vi "run.vi"(8 "error in (no error)":errorcluster, 11 "DL090216Display in":refnum<class "DisplayDL090216.lvclass">) -> (0 "error out":errorcluster, 3 "DL090216Display out":refnum<class "DisplayDL090216.lvclass">)   [LabVIEW 2010, in "DisplayDL090216.lvclass"]
uses:
  DisplayDL090216.lvclass
  common/clusters/range_offset_cluster.ctl
  common/enumerations/channel_display_colour_enum.ctl
  individual_channel_cluster.ctl
  main/labview_source/controls/undock_button.ctl
  action_enum.ctl
  <vilib>/vision/Image Controls.llb/IMAQ Image.ctl
  DisplayDL090216.lvclass/DisplayDL090216.ctl
  ImageProcessor/ImageProcessorDL090216RangeOffset/ImageProcessorDL090216RangeOffset/ImageProcessorDL090216RangeOffset.lvclass
  GenericDisplay/GenericDisplay/GenericDisplay.lvclass
  ImageProcessor/GenericImageProcessor/GenericImageProcessor/GenericImageProcessor.lvclass
  common/classes/Image/Image/colour_enum.ctl
  common/classes/ErrorController/ErrorController/class_data.vi
  common/classes/Image/Image/Image.lvclass
  common/classes/GenericComponent/GenericComponent/GenericComponent.lvclass
  common/classes/ErrorController/ErrorController/ErrorController.lvclass
panel:
  in  "button:undock_main_window":T1
  in  "button:undock":T1
  in  "button_configure":bool
  in  "channel tab":enum32{"Individual channels", "Debug"}(tab)
  in  "channel 3":T2
  in  "channel 2":T2
  in  "channel 1":T2
  out "statechart error":errorcluster
  out "event handling loop error":errorcluster
  out "first image received?":bool
  out "event handling loop counter":i32
  out "statemachine loop counter":i32
  out "current action":T4
  out "last trigger":T4
  in  "Tab Control":enum32{"Image", "Performance", "Extra"}(tab)=enum."Performance"
  in  "master range and offset":T5={"range"=0.5, "offset"=0.5} {"offset" min=0.0 max=1.0 step=0.0010000000474974513 scale=0.0..1.0; "range" min=0.0 max=1.0 step=0.0010000000474974513 scale=0.0..1.0}
  in  "optimise":bool
  in  "adjust range/offset button":bool
  in  "channel colours":T6[](array[typedef])=[enum."red", enum."green", enum."blue", enum."red"]
  in  "elements in queue":i32
  in  "maximum resolution":i32=256 min=0 max=512
  in  "maximum update rate":dbl[unit]=10.0 min=0.0
  in  "button:show_histogram?":bool caption="show histogram"
  in  "x scaling":dbl(slide)=1.0 min=0.05 max=20.0 step=0.01 scale=0.05..20.0
  in  "rotated by":dbl[unit]
  in  "enable x middle line?":bool
  in  "enable y middle line?":bool
  in  "enable scale bar?":bool
  in  "flipped?":bool
  in  "zero rotation button":bool
  in  "averaging":i32=1 min=1 max=100 step=1
  in  "stop":bool
  out "main display":T3(plugin-control)
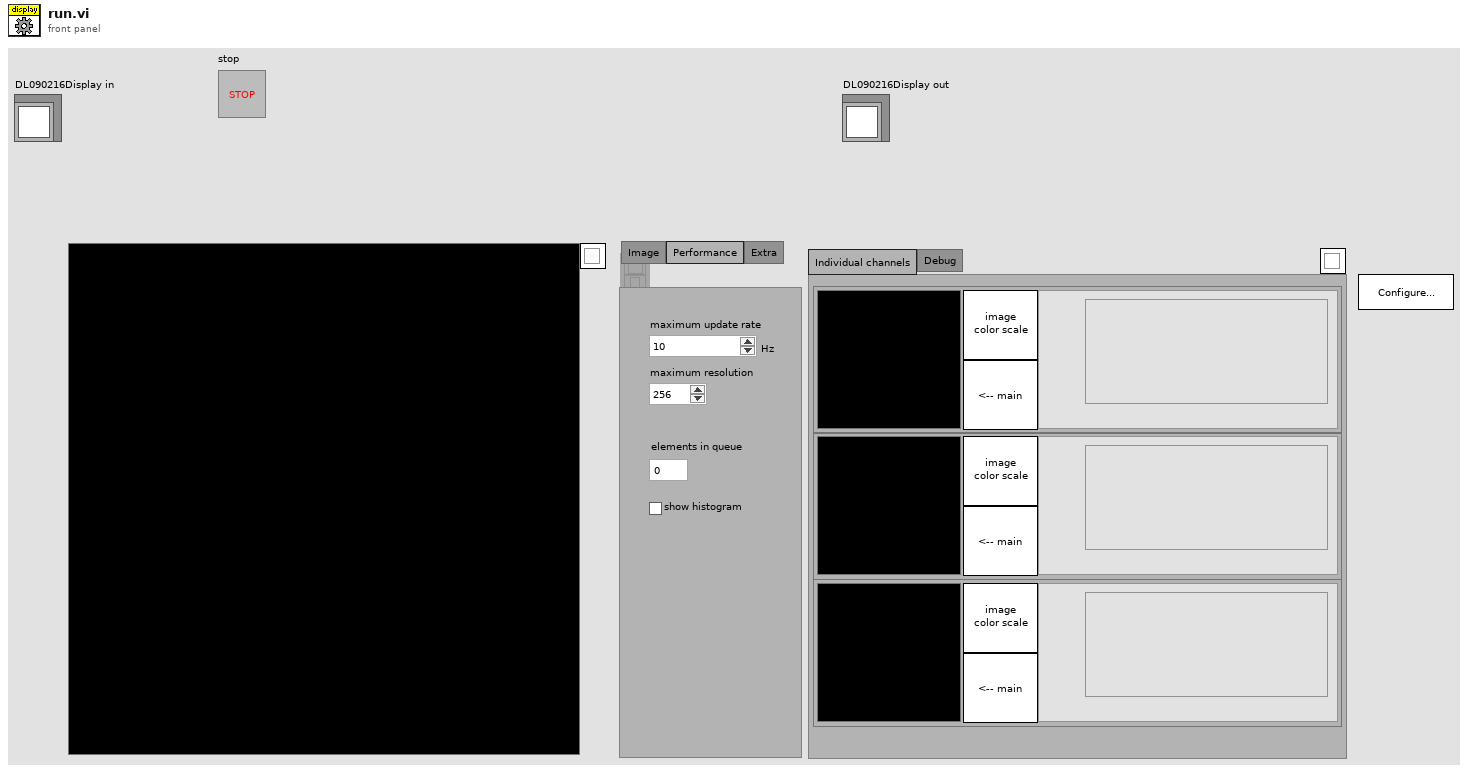
[diagram p1: front panel]
types:
  T1 = typedef "undock_button.ctl" = bool
  T2 = typedef "DisplayDL090216.lvclass/individual_channel_cluster.ctl" = cluster{"Image":T3, "histogram out":cluster{i32, u32}[], "button:color scale":bool, "button:set as main image":bool}
  T3 = typedef "IMAQ Image.ctl" = refnum<image>
  T4 = typedef "DisplayDL090216.lvclass/action_enum.ctl" = enum16{"NULL", "initialise", "experiment started", "experiment stopped", "terminate", "fetch", "process", "display", "register as observer"}
  T5 = typedef "range_offset_cluster.ctl" = cluster{"range":dbl, "offset":dbl}
  T6 = typedef "channel_display_colour_enum.ctl" = enum16{"none", "red", "green", "blue", "grey scale", "custom"}
  T7 = typedef "main_trigger_enum.ctl" = enum16{"NULL", "initialise", "terminate", "start", "stop", "change objective", "change experimentController", "change imagingMode", "save notebook", "started saving", "finished saving", "expCtr ready", "expCtr missing", "imgMd ready", "imgMd missing", "scanHd ready", "scanHd missing", "DAQ ready", "DAQ missing", "imgAsm ready", "imgAsm missing", "dataColl ready", "dataColl missing", "display ready", "display missing", "analysr ready", "analysr missing", "instrmnt ready", "instrmnt missing", "stimltr ready", "stimltr missing", "stage ready", "stage missing"}
  T8 = enum8{"Enabled", "Disabled", "Disabled and Grayed Out"}
  T9 = typedef "Image.lvclass/colour_enum.ctl" = enum16{"none", "red", "green", "blue", "grey scale", "custom"}
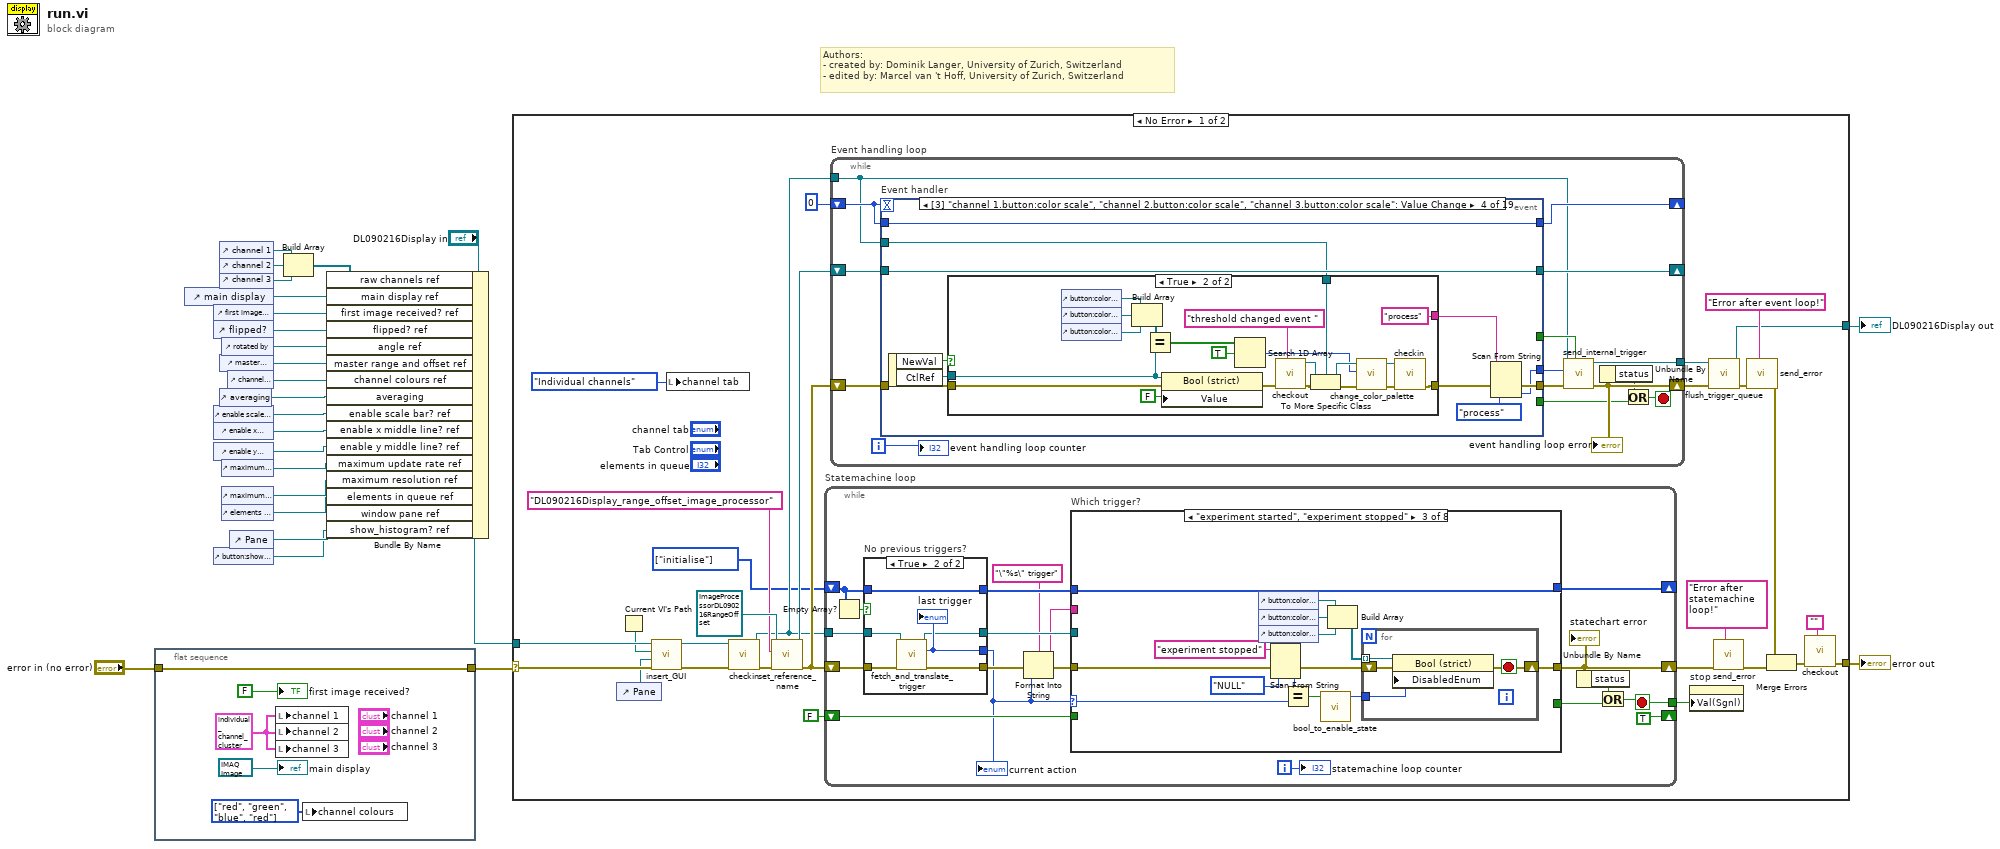
[diagram p0: block diagram]
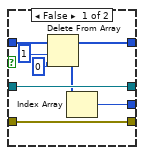
[diagram p2: hidden frame]
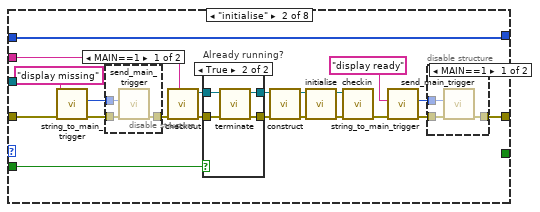
[diagram p4: hidden frame]
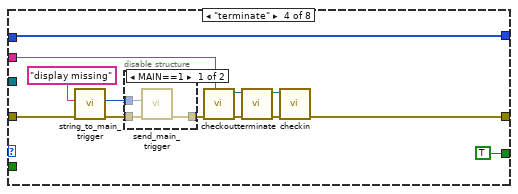
[diagram p8: hidden frame]
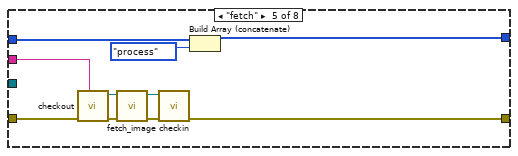
[diagram p10: hidden frame]
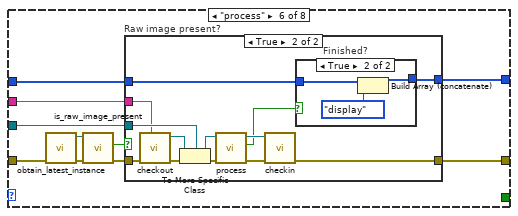
[diagram p11: hidden frame]
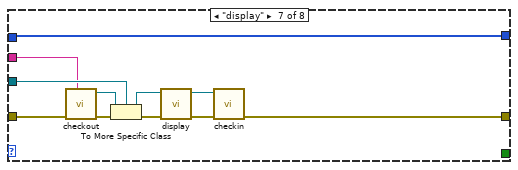
[diagram p14: hidden frame]
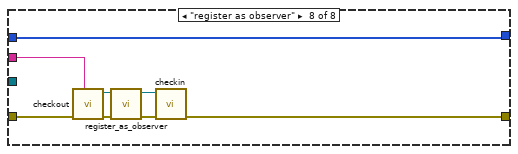
[diagram p15: hidden frame]
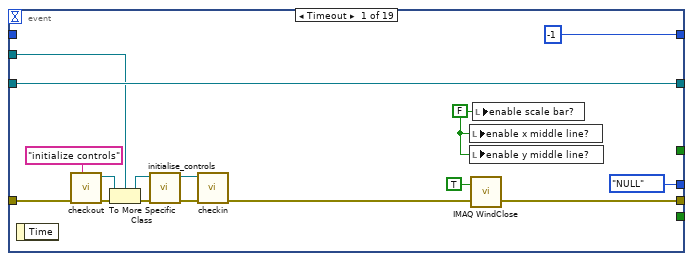
[diagram p16: hidden frame]
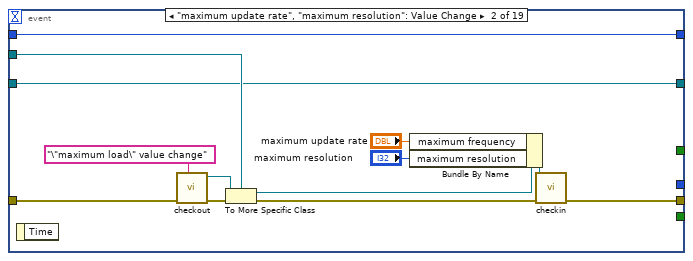
[diagram p17: hidden frame]
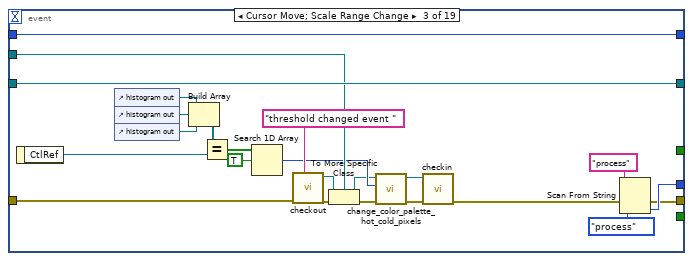
[diagram p18: hidden frame]
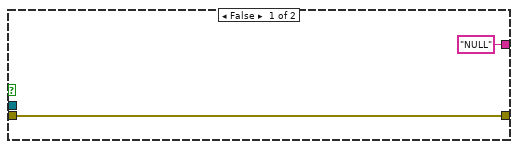
[diagram p19: hidden frame]
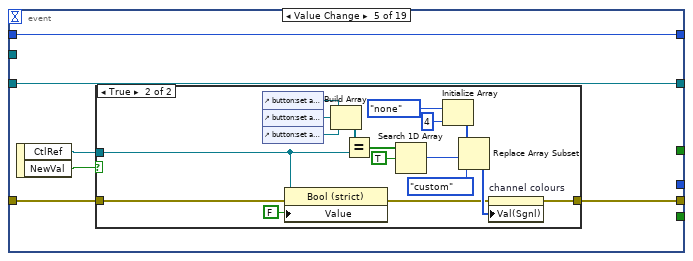
[diagram p20: hidden frame]
diagram:
  # "Authors: \n- created by: Dominik Langer, University of Zurich, Switzerland\n- edited by: Marcel van 't Hoff, University of Zurich, Switzerland"
  n1 = flat-sequence {
    tunnel: "error in (no error)" -> [w30]
    tunnel: [w30] -> w6
    frame #0 {
      w26 = T6[] [enum."red", enum."green", enum."blue", enum."red"] items=["none", "red", "green", "blue", "grey scale", "custom"] ("channel colours")
      w27 = T2 {"Image"=refnum, "histogram out"=[], "button:color scale"=FALSE, "button:set as main image"=FALSE} ("channel 1")
      n2 = local write "channel 1"(w27) -> ()
      n3 = local write "channel 2"(w27) -> ()
      n4 = local write "channel 3"(w27) -> ()
      n5 = local write "channel colours"(w26) -> ()
      "first image received?" <- FALSE
      "main display" <- T3 refnum ("main display")
    }
  }
  n6 = control-ref of="main display"() -> (w21:refnum<vi>)
  n7 = control-ref of="first image received?"() -> (w3:refnum<vi>)
  n8 = control-ref of="flipped?"() -> (w20:refnum<vi>)
  n9 = control-ref of="enable scale bar?"() -> (w16:refnum<vi>)
  n10 = control-ref of="enable x middle line?"() -> (w15:refnum<vi>)
  n11 = control-ref of="enable y middle line?"() -> (w14:refnum<vi>)
  n12 = control-ref of="button:show_histogram?"() -> (w2:refnum<vi>)
  n13 = control-ref of="channel 1"() -> (w8:refnum<vi>)
  n14 = control-ref of="channel 2"() -> (w9:refnum<vi>)
  n15 = control-ref of="channel 3"() -> (w10:refnum<vi>)
  n16 = control-ref of="master range and offset"() -> (w17:refnum<vi>)
  n17 = control-ref of="averaging"() -> (w1:refnum<vi>)
  n18 = control-ref of="rotated by"() -> (w19:refnum<vi>)
  n19 = control-ref of="maximum update rate"() -> (w5:refnum<vi>)
  n20 = control-ref of="maximum resolution"() -> (w13:refnum<vi>)
  n21 = control-ref of="elements in queue"() -> (w12:refnum<vi>)
  n22 = control-ref of="channel colours"() -> (w18:refnum<vi>)
  n23 = control-ref of="Pane"() -> (w11:refnum<vi>)
  n24 = Build Array(w8, w9, w10) -> (w4:refnum<vi>[])
  n25 = Bundle By Name(cluster="DL090216Display in", "raw channels ref"=w4, "main display ref"=w21, "first image received? ref"=w3, "flipped? ref"=w20, "angle ref"=w19, "master range and offset ref"=w17, "channel colours ref"=w18, "averaging"=w1, "enable scale bar? ref"=w16, "enable x middle line? ref"=w15, "enable y middle line? ref"=w14, "maximum update rate ref"=w5, "maximum resolution ref"=w13, "elements in queue ref"=w12, "window pane ref"=w11, "show_histogram? ref"=w2) -> (w22:refnum<class "DisplayDL090216.lvclass">)
  n26 = case shown="No Error" w6 {
    selector: w6 -> [w51 w575]
    tunnel: [w43 w575] -> w25
    tunnel: [w41 w574] -> w24
    tunnel: w22 -> [w50 w574]
    frame No Error {
      w34 = T4[] [enum."initialise"] items=["NULL", "initialise", "experiment started", "experiment stopped", "terminate", "fetch", "process", "display", "register as observer"]
      n27 = control-ref of="Pane"() -> (w48:refnum<vi>)
      n28 = Current VI's Path() -> (path=w49:path)
      n29 = call-dynamic "insert_GUI.vi"("error in (no error)"=w51, "Pane"=w48, "VI path"=w49, "GenericComponent in"=w50) -> ("error out"=w33:errorcluster, "GenericComponent out"=w36:refnum<class "DisplayDL090216.lvclass">)  [unwired: 6 in]
      n30 = local write "channel tab"(enum32{"Individual channels", "Debug"}."Individual channels" ("channel tab")) -> ()
      n31 = call-dynamic "checkin.vi"("error in (no error)"=w33, "GenericDisplay in"=w36) -> ("error out"=w53:errorcluster, "GenericDisplay out"=w37:refnum<class "DisplayDL090216.lvclass">)  [unwired: 8 in]
      n32 = call "set_reference_name.vi"("error in (no error)"=w53, "reference name"="DL090216Display_range_offset_image_processor", "GenericPlugin.lvclass in"=refnum<class "ImageProcessorDL090216RangeOffset.lvclass"> refnum ("ImageProcessorDL090216RangeOffset.lvclass")) -> ("error out"=w38:errorcluster, "GenericPlugin.lvclass out"=w52:refnum<class "ImageProcessorDL090216RangeOffset.lvclass">)  [unwired: 7 in]
      n33 = while "Statemachine loop" {
        shift-right: [w75] -> w32
        shift-left: w38 -> [w76]
        tunnel: [w72] -> w57
        tunnel: w37 -> [w77]
        shift-right: [w71] -> _
        shift-left: w34 -> [w68]
        shift-right: [TRUE] -> _
        shift-left: FALSE -> [w66]
        i -> [w78]
        stop <- w72 stop-if-true
        n34 = Empty Array?(array=w68) -> (empty?=w67:bool)
        n35 = case "No previous triggers?" shown="True" w67 {
          tunnel: w77 -> [w85 w92]
          tunnel: w76 -> [w86 w91]
          tunnel: [w86 w90] -> w64
          tunnel: [w79 w89] -> w63
          tunnel: w68 -> [w84 w88]
          tunnel: [w81 w88] -> w70
          tunnel: [w85 w87] -> w69
          frame False {
            n36 = Delete From Array(array=w84, length=1, index=0) -> (deleted portion=w80:T4[], array with subset deleted=w81:T4[])
            n37 = Index Array(array=w80) -> (element=w79:T4)  [unwired: 1 in]
          }
          frame True {
            n38 = call-dynamic "fetch_and_translate_trigger.vi"("error in (no error)"=w91, "DisplayDL090216 in"=w92) -> ("error out"=w90:errorcluster, "internal trigger"=w89:T4, "DisplayDL090216 out"=w87:refnum<class "DisplayDL090216.lvclass">)  [unwired: 6 in, 1 out]
            "last trigger" <- w89
          }
        }
        "current action" <- w63
        n39 = Format Into String(format string="\"%s\" trigger", error in=w64, w63) -> (resulting string=w61:string, error out=w62:errorcluster)  [unwired: 1 in]
        n40 = case "Which trigger?" shown="\"experiment started\", \"experiment stopped\"" w63 {
          selector: w63 -> [_ _ w137 _ _ _ _ _]
          tunnel: w62 -> [w94 w97 w131 w151 w170 w180 w208 w218]
          tunnel: [w94 w111 w138 w157 w169 w177 w207 w217] -> w75
          tunnel: [_ _ _ TRUE _ _ _ _] -> w74
          tunnel: [w93 w110 w143 w153 w167 w183 w206 w216] -> w71
          tunnel: w70 -> [w93 w110 w143 w153 w166 w184 w206 w216]
          tunnel: w69 -> [_ _ _ _ _ w178 w205 _]
          tunnel: w66 -> [_ w105 _ _ _ _ _ _]
          tunnel: w61 -> [_ w104 _ w152 w165 w175 w204 w215]
          frame "NULL", Default {
          }
          frame "initialise" {
            n41 = call "string_to_main_trigger.vi"("error in (no error)"=w97, "trigger string"="display missing") -> ("error out"=w99:errorcluster, "main trigger"=w98:T7)  [unwired: 8 in]
            n42 = disable-structure shown="MAIN==1" {
              disable-tunnel: w99 -> [w118 w119]
              disable-tunnel: [w117 w119] -> w96
              disable-tunnel: w98 -> [w116 _]
              frame condition #0 {
                n43 = call "send_main_trigger.vi"("error in (no error)"=w118, "trigger"=w116) -> ("error out"=w117:errorcluster)  [unwired: 9 in]
              }
              frame condition #1 (active) {
              }
            }
            n44 = call "checkout.vi"("locked by?"=w104, "error in (no error)"=w96) -> ("error out"=w109:errorcluster, "GenericDisplay out"=w108:refnum<class "GenericDisplay.lvclass">)  [unwired: 8 out]
            n45 = case "Already running?" shown="True" w105 {
              tunnel: w109 -> [w124 w129]
              tunnel: w108 -> [w125 w128]
              tunnel: [w125 w127] -> w107
              tunnel: [w124 w126] -> w106
              frame False {
              }
              frame True {
                n46 = call-dynamic "terminate.vi"("error in (no error)"=w129, "GenericPlugin in"=w128) -> ("error out"=w126:errorcluster, "GenericPlugin out"=w127:refnum<class "GenericDisplay.lvclass">)  [unwired: 8 in]
              }
            }
            n47 = call-dynamic "construct.vi"("error in (no error)"=w106, "GenericPlugin in"=w107) -> ("error out"=w115:errorcluster, "GenericPlugin out"=w114:refnum<class "GenericDisplay.lvclass">)  [unwired: 2 in, 6 out]
            n48 = call-dynamic "initialise.vi"("error in (no error)"=w115, "GenericPlugin in"=w114) -> ("error out"=w113:errorcluster, "GenericPlugin out"=w112:refnum<class "GenericDisplay.lvclass">)  [unwired: 8 out]
            n49 = call-dynamic "checkin.vi"("error in (no error)"=w113, "GenericDisplay in"=w112) -> ("error out"=w101:errorcluster)  [unwired: 8 in, 1 out]
            n50 = call "string_to_main_trigger.vi"("error in (no error)"=w101, "trigger string"="display ready") -> ("error out"=w100:errorcluster, "main trigger"=w102:T7)  [unwired: 8 in]
            n51 = disable-structure shown="MAIN==1" {
              disable-tunnel: w100 -> [w122 w123]
              disable-tunnel: [w121 w123] -> w111
              disable-tunnel: w102 -> [w120 _]
              frame condition #0 {
                n52 = call "send_main_trigger.vi"("error in (no error)"=w122, "trigger"=w120) -> ("error out"=w121:errorcluster)  [unwired: 9 in]
              }
              frame condition #1 (active) {
              }
            }
          }
          frame "experiment started", "experiment stopped" {
            n53 = control-ref of="button:color scale"() -> (w140:refnum<vi>)
            n54 = control-ref of="button:color scale"() -> (w141:refnum<vi>)
            n55 = control-ref of="button:color scale"() -> (w142:refnum<vi>)
            n56 = Scan From String(input string="experiment stopped", error in=w131, default 1=action_enum."NULL" ("y")) -> (error out=w135:errorcluster, output 1=w133:T4)  [unwired: 2 in, 2 out]
            n57 = Equal?(x=w133, y=w137) -> (x = y?=w130:bool)
            n58 = call "bool_to_enable_state.vi"("boolean in"=w130) -> ("enabled status out"=w132:T8)  [unwired: 4 in]
            n59 = Build Array(w140, w141, w142) -> (w139:refnum<vi>[])
            n60 = for {
              tunnel: w139 -> [w147] mode=indexing
              shift-right: [w145] -> w138
              shift-left: w135 -> [w146]
              tunnel: w132 -> [w144]
              stop <- w145 stop-if-true
              n61 = property class="Bool (strict)"(reference=w147, error in=w146, "DisabledEnum"=w144) -> (error out=w145:errorcluster)  [unwired: 1 out]
            }
          }
          frame "terminate" {
            n62 = call "string_to_main_trigger.vi"("error in (no error)"=w151, "trigger string"="display missing") -> ("error out"=w150:errorcluster, "main trigger"=w148:T7)  [unwired: 8 in]
            n63 = disable-structure shown="MAIN==1" {
              disable-tunnel: w150 -> [w163 w164]
              disable-tunnel: [w162 w164] -> w154
              disable-tunnel: w148 -> [w161 _]
              frame condition #0 {
                n64 = call "send_main_trigger.vi"("error in (no error)"=w163, "trigger"=w161) -> ("error out"=w162:errorcluster)  [unwired: 9 in]
              }
              frame condition #1 (active) {
              }
            }
            n65 = call "checkout.vi"("locked by?"=w152, "error in (no error)"=w154) -> ("error out"=w156:errorcluster, "GenericDisplay out"=w158:refnum<class "GenericDisplay.lvclass">)  [unwired: 8 out]
            n66 = call-dynamic "terminate.vi"("error in (no error)"=w156, "GenericPlugin in"=w158) -> ("error out"=w155:errorcluster, "GenericPlugin out"=w159:refnum<class "GenericDisplay.lvclass">)  [unwired: 8 out]
            n67 = call-dynamic "checkin.vi"("error in (no error)"=w155, "GenericDisplay in"=w159) -> ("error out"=w157:errorcluster)  [unwired: 8 in, 1 out]
          }
          frame "fetch" {
            n68 = call "checkout.vi"("locked by?"=w165, "error in (no error)"=w170) -> ("error out"=w173:errorcluster, "GenericDisplay out"=w172:refnum<class "GenericDisplay.lvclass">)  [unwired: 8 out]
            n69 = call-dynamic "fetch_image.vi"("error in (no error)"=w173, "GenericToplevelComponent in"=w172) -> ("error out"=w174:errorcluster, "GenericToplevelComponent out"=w171:refnum<class "GenericDisplay.lvclass">)  [unwired: 4 in, 4 out]
            n70 = call-dynamic "checkin.vi"("error in (no error)"=w174, "GenericDisplay in"=w171) -> ("error out"=w169:errorcluster)  [unwired: 8 in, 1 out]
            n71 = Build Array (concatenate)(w166, action_enum."process" ("last trigger")) -> (w167:T4[])
          }
          frame "process" {
            n72 = call "obtain_latest_instance.vi"("error in (no error)"=w180) -> ("error out"=w182:errorcluster, "GenericDisplay out"=w181:refnum<class "GenericDisplay.lvclass">)  [unwired: 1 in, 8 out]
            n73 = call-dynamic "is_raw_image_present.vi"("error in (no error)"=w182, "GenericDisplay in"=w181) -> ("error out"=w179:errorcluster, "raw image present?"=w176:bool)  [unwired: 8 out]
            n74 = case "Raw image present?" shown="True" w176 {
              tunnel: w184 -> [w186 w199]
              tunnel: [w186 w198] -> w183
              tunnel: w179 -> [w185 w192]
              tunnel: w178 -> [_ w191]
              tunnel: [w185 w189] -> w177
              tunnel: w175 -> [_ w188]
              frame False {
              }
              frame True {
                n75 = call "checkout.vi"("locked by?"=w188, "error in (no error)"=w192) -> ("error out"=w197:errorcluster, "GenericDisplay out"=w196:refnum<class "GenericDisplay.lvclass">)  [unwired: 8 out]
                n76 = To More Specific Class(target class=w191, reference=w196, error in=w197) -> (specific class reference=w190:refnum<class "DisplayDL090216.lvclass">, error out=w195:errorcluster)
                n77 = call-dynamic "process.vi"("error in (no error)"=w195, "DL090216Display in"=w190) -> ("error out"=w194:errorcluster, "finished?"=w187:bool, "DL090216Display out"=w193:refnum<class "DisplayDL090216.lvclass">)  [unwired: 7 out]
                n78 = call-dynamic "checkin.vi"("error in (no error)"=w194, "GenericDisplay in"=w193) -> ("error out"=w189:errorcluster)  [unwired: 8 in, 1 out]
                n79 = case "Finished?" shown="True" w187 {
                  tunnel: w199 -> [w200 w203]
                  tunnel: [w200 w201] -> w198
                  frame False {
                  }
                  frame True {
                    n80 = Build Array (concatenate)(w203, action_enum."display" ("last trigger")) -> (w201:T4[])
                  }
                }
              }
            }
          }
          frame "display" {
            n81 = call "checkout.vi"("locked by?"=w204, "error in (no error)"=w208) -> ("error out"=w214:errorcluster, "GenericDisplay out"=w213:refnum<class "GenericDisplay.lvclass">)  [unwired: 8 out]
            n82 = To More Specific Class(target class=w205, reference=w213, error in=w214) -> (specific class reference=w209:refnum<class "DisplayDL090216.lvclass">, error out=w210:errorcluster)
            n83 = call-dynamic "display.vi"("error in (no error)"=w210, "DL090216Display in"=w209) -> ("error out"=w212:errorcluster, "DL090216Display out"=w211:refnum<class "DisplayDL090216.lvclass">)  [unwired: 8 out]
            n84 = call-dynamic "checkin.vi"("error in (no error)"=w212, "GenericDisplay in"=w211) -> ("error out"=w207:errorcluster)  [unwired: 8 in, 1 out]
          }
          frame "register as observer" {
            n85 = call "checkout.vi"("locked by?"=w215, "error in (no error)"=w218) -> ("error out"=w220:errorcluster, "GenericDisplay out"=w222:refnum<class "GenericDisplay.lvclass">)  [unwired: 8 in]
            n86 = call-dynamic "register_as_observer.vi"("error in (no error)"=w220, "GenericToplevelComponent in"=w222) -> ("error out"=w219:errorcluster, "GenericToplevelComponent out"=w221:refnum<class "GenericDisplay.lvclass">)  [unwired: 8 in]
            n87 = call-dynamic "checkin.vi"("error in (no error)"=w219, "GenericDisplay in"=w221) -> ("error out"=w217:errorcluster)  [unwired: 8 in, 1 out]
          }
        }
        "statechart error" <- w75
        n88 = Unbundle By Name(w75) -> ("status"=w73:bool)
        n89 = Or(x=w73, y=w74) -> (x .or. y?=w72:bool)
        "statemachine loop counter" <- w78
      }
      n90 = while "Event handling loop" {
        shift-right: [w227] -> w42
        shift-left: w38 -> [w237]
        shift-right: [w235] -> _
        shift-left: 0 -> [w236]
        shift-right: [w233] -> _
        shift-left: w52 -> [w232]
        tunnel: w37 -> [w228]
        tunnel: [w230] -> w40
        i -> [w234]
        stop <- w224 stop-if-true
        n91 = event "Event handler" shown="[3] \"channel 1.button:color scale\", \"channel 2.button:color scale\", \"channel 3.button:color scale\": Value Change" {
          selector: _ -> [_ _ _ _ _ _ _ _ _ _ _ _ _ _ _ _ _ _ _]
          dyn-events: _ -> [_ _ _ _ _ _ _ _ _ _ _ _ _ _ _ _ _ _ _]
          timeout: w236 -> [_ _ _ _ _ _ _ _ _ _ _ _ _ _ _ _ _ _ _]
          tunnel: w237 -> [w249 w264 w288 w297 w328 w364 w378 w384 w401 w420 w426 w446 w453 w474 w500 w516 w521 w555 w568]
          tunnel: [w240 w263 w267 w293 w327 w349 w374 w383 w392 w419 w425 w431 w452 w465 w488 w510 w524 w541 w561] -> w231
          tunnel: [-1 w266 w290 w301 w330 w361 w380 w387 w403 w423 w429 w450 w463 w486 w504 w518 w539 w559 w573] -> w235
          tunnel: w236 -> [_ w266 w290 w301 w330 w361 w380 w387 w403 w423 w429 w450 w463 w486 w504 w518 w539 w559 w573]
          tunnel: [_ _ _ _ _ _ _ _ _ _ TRUE _ _ _ _ _ _ _ _] -> w225
          tunnel: w228 -> [w245 w259 w287 w299 _ w359 w371 w385 w398 _ _ w445 w458 w475 _ w508 w538 w554 w571]
          tunnel: [w251 w255 w289 w300 w329 w366 w379 w386 w402 w422 w427 w435 w455 w476 w493 w509 w528 w545 w565] -> w233
          tunnel: w232 -> [w251 w255 w289 w300 w329 w366 w379 w386 w402 w422 w427 w435 w454 w476 w493 w509 w528 w545 w565]
          tunnel: [_ _ _ _ _ _ _ _ _ _ _ _ TRUE _ _ _ _ _ _] -> w229
          tunnel: [action_enum."NULL" ("trigger") _ w269 w292 _ w351 _ _ _ _ _ w430 _ w464 w487 _ w523 w540 w560] -> w223
          event Timeout {
            w252 = FALSE
            n92 = event-data() -> ()  [unwired: 2 out]
            n93 = call "checkout.vi"("locked by?"="initialize controls", "error in (no error)"=w249) -> ("error out"=w250:errorcluster, "GenericDisplay out"=w246:refnum<class "GenericDisplay.lvclass">)  [unwired: 8 out]
            n94 = To More Specific Class(target class=w245, reference=w246, error in=w250) -> (specific class reference=w244:refnum<class "DisplayDL090216.lvclass">, error out=w248:errorcluster)
            n95 = call-dynamic "initialise_controls.vi"("error in (no error)"=w248, "DL090216Display in"=w244) -> ("error out"=w247:errorcluster, "DL090216Display out"=w243:refnum<class "DisplayDL090216.lvclass">)  [unwired: 8 out]
            n96 = call-dynamic "checkin.vi"("error in (no error)"=w247, "GenericDisplay in"=w243) -> ("error out"=w241:errorcluster)  [unwired: 8 in, 1 out]
            n97 = local write "enable x middle line?"(w252) -> ()
            n98 = local write "enable y middle line?"(w252) -> ()
            n99 = call "IMAQ WindClose"("Close All Windows (False)"=TRUE, "error in (no error)"=w241) -> ("error out"=w240:errorcluster)  [unwired: 4 in]
            n100 = local write "enable scale bar?"(w252) -> ()
          }
          event "maximum update rate", "maximum resolution": Value Change {
            n101 = event-data() -> ()  [unwired: 2 out]
            n102 = call "checkout.vi"("locked by?"="\"maximum load\" value change", "error in (no error)"=w264) -> ("error out"=w262:errorcluster, "GenericDisplay out"=w260:refnum<class "GenericDisplay.lvclass">)  [unwired: 8 in]
            n103 = To More Specific Class(target class=w259, reference=w260, error in=w262) -> (specific class reference=w258:refnum<class "DisplayDL090216.lvclass">, error out=w261:errorcluster)
            n104 = Bundle By Name(cluster=w258, "maximum frequency"="maximum update rate", "maximum resolution"="maximum resolution") -> (w257:refnum<class "DisplayDL090216.lvclass">)
            n105 = call-dynamic "checkin.vi"("error in (no error)"=w261, "GenericDisplay in"=w257) -> ("error out"=w263:errorcluster)  [unwired: 8 in, 1 out]
          }
          event Cursor Move; Scale Range Change {
            n106 = event-data() -> ("CtlRef"=w286:refnum<vi>)  [unwired: 1 out]
            n107 = control-ref of="histogram out"() -> (w282:refnum<vi>)
            n108 = control-ref of="histogram out"() -> (w281:refnum<vi>)
            n109 = control-ref of="histogram out"() -> (w280:refnum<vi>)
            n110 = Build Array(w282, w281, w280) -> (w279:refnum<vi>[])
            n111 = Equal?(x=w279, y=w286) -> (x = y?=w278:bool[])
            n112 = Search 1D Array(1D array=w278, element=TRUE) -> (index of element=w276:i32)  [unwired: 1 in]
            n113 = call "checkout.vi"("locked by?"="threshold changed event ", "error in (no error)"=w288) -> ("error out"=w285:errorcluster, "GenericDisplay out"=w284:refnum<class "GenericDisplay.lvclass">)  [unwired: 8 out]
            n114 = To More Specific Class(target class=w287, reference=w284, error in=w285) -> (specific class reference=w275:refnum<class "DisplayDL090216.lvclass">, error out=w273:errorcluster)
            n115 = call-dynamic "change_color_palette_hot_cold_pixels.vi"("error in (no error)"=w273, "raw channel index"=w276, "DisplayDL090216 in"=w275) -> ("error out"=w272:errorcluster, "DisplayDL090216 out"=w274:refnum<class "DisplayDL090216.lvclass">)  [unwired: 7 in]
            n116 = call-dynamic "checkin.vi"("error in (no error)"=w272, "GenericDisplay in"=w274) -> ("error out"=w268:errorcluster)  [unwired: 8 in, 1 out]
            n117 = Scan From String(input string="process", error in=w268, default 1=action_enum."process" ("trigger")) -> (error out=w267:errorcluster, output 1=w269:T4)  [unwired: 2 in, 2 out]
          }
          event Value Change {
            n118 = event-data() -> ("NewVal"=w296:bool, "CtlRef"=w298:refnum<vi>)  [unwired: 1 out]
            n119 = case shown="True" w296 {
              tunnel: [w303 w324] -> w294
              tunnel: w299 -> [_ w323]
              tunnel: w298 -> [_ w308]
              tunnel: w297 -> [w303 w307]
              tunnel: ["NULL" "process"] -> w291
              frame False {
              }
              frame True {
                n120 = control-ref of="button:color scale"() -> (w319:refnum<vi>)
                n121 = control-ref of="button:color scale"() -> (w318:refnum<vi>)
                n122 = control-ref of="button:color scale"() -> (w317:refnum<vi>)
                n123 = Build Array(w319, w318, w317) -> (w316:refnum<vi>[])
                n124 = Equal?(x=w316, y=w308) -> (x = y?=w315:bool[])
                n125 = property class="Bool (strict)"(reference=w308, error in=w307, "Value"=FALSE) -> (error out=w306:errorcluster)  [unwired: 1 out]
                n126 = Search 1D Array(1D array=w315, element=TRUE) -> (index of element=w309:i32)  [unwired: 1 in]
                n127 = call "checkout.vi"("locked by?"="threshold changed event ", "error in (no error)"=w306) -> ("error out"=w322:errorcluster, "GenericDisplay out"=w321:refnum<class "GenericDisplay.lvclass">)  [unwired: 8 out]
                n128 = To More Specific Class(target class=w323, reference=w321, error in=w322) -> (specific class reference=w313:refnum<class "DisplayDL090216.lvclass">, error out=w311:errorcluster)
                n129 = call-dynamic "change_color_palette.vi"("error in (no error)"=w311, "raw channel index"=w309, "DisplayDL090216 in"=w313) -> ("error out"=w310:errorcluster, "DisplayDL090216 out"=w312:refnum<class "DisplayDL090216.lvclass">)  [unwired: 7 in]
                n130 = call-dynamic "checkin.vi"("error in (no error)"=w310, "GenericDisplay in"=w312) -> ("error out"=w324:errorcluster)  [unwired: 8 in, 1 out]
              }
            }
            n131 = Scan From String(input string=w291, error in=w294, default 1=action_enum."process" ("trigger")) -> (error out=w293:errorcluster, output 1=w292:T4)  [unwired: 2 in, 2 out]
          }
          event Value Change {
            n132 = event-data() -> ("CtlRef"=w326:refnum<vi>, "NewVal"=w325:bool)  [unwired: 1 out]
            n133 = case shown="True" w325 {
              tunnel: w328 -> [w331 w334]
              tunnel: [w331 w348] -> w327
              tunnel: w326 -> [_ w335]
              frame False {
              }
              frame True {
                n134 = control-ref of="button:set as main image"() -> (w346:refnum<vi>)
                n135 = control-ref of="button:set as main image"() -> (w347:refnum<vi>)
                n136 = control-ref of="button:set as main image"() -> (w345:refnum<vi>)
                n137 = property class="Bool (strict)"(reference=w335, error in=w334, "Value"=FALSE) -> (error out=w333:errorcluster)  [unwired: 1 out]
                n138 = Build Array(w346, w347, w345) -> (w344:refnum<vi>[])
                n139 = Equal?(x=w344, y=w335) -> (x = y?=w343:bool[])
                n140 = Search 1D Array(1D array=w343, element=TRUE) -> (index of element=w338:i32)  [unwired: 1 in]
                n141 = Initialize Array(channel_display_colour_enum."none" ("channel x"), 4 ("element")) -> (w339:T6[])
                n142 = Replace Array Subset(array=w339, new element=channel_display_colour_enum."custom" ("new element/subarray"), index=w338) -> (w336:T6[])
                n143 = property on="channel colours" class="Arr (strict)"(error in=w333, "Val(Sgnl)"=w336) -> (error out=w348:errorcluster)  [unwired: 1 in, 1 out]
              }
            }
          }
          event "button_configure": Value Change {
            n144 = event-data() -> ()  [unwired: 4 out]
            n145 = call "checkout.vi"("locked by?"=" \"button_configure\" value change" ("string"), "error in (no error)"=w364) -> ("error out"=w365:errorcluster, "GenericDisplay out"=w363:refnum<class "GenericDisplay.lvclass">)  [unwired: 8 out]
            n146 = call-dynamic "configure.vi"("error in (no error)"=w365, "GenericPlugin in"=w363) -> ("error out"=w355:errorcluster, "GenericPlugin out"=w360:refnum<class "GenericDisplay.lvclass">)  [unwired: 8 in]
            n147 = To More Specific Class(target class=w359, reference=w360, error in=w355) -> (specific class reference=w358:refnum<class "DisplayDL090216.lvclass">, error out=w357:errorcluster)
            n148 = call-dynamic "set_histogram_enabled.vi"("error in (no error)"=w357, "DisplayDL090216 in"=w358) -> ("error out"=w354:errorcluster, "DisplayDL090216 out"=w356:refnum<class "DisplayDL090216.lvclass">)  [unwired: 8 in]
            n149 = call-dynamic "checkin.vi"("error in (no error)"=w354, "GenericDisplay in"=w356) -> ("error out"=w350:errorcluster)  [unwired: 8 in, 1 out]
            n150 = Scan From String(input string="initialise", error in=w350, default 1=action_enum."process" ("trigger")) -> (error out=w349:errorcluster, output 1=w351:T4)  [unwired: 2 in, 2 out]
          }
          event "button:show_histogram?": Value Change {
            n151 = event-data() -> ()  [unwired: 4 out]
            n152 = call "checkout.vi"("locked by?"=" \"button_histogram?\" value change" ("string"), "error in (no error)"=w378) -> ("error out"=w376:errorcluster, "GenericDisplay out"=w372:refnum<class "GenericDisplay.lvclass">)  [unwired: 8 out]
            n153 = To More Specific Class(target class=w371, reference=w372, error in=w376) -> (specific class reference=w370:refnum<class "DisplayDL090216.lvclass">, error out=w377:errorcluster)
            n154 = Bundle By Name(cluster=w370, "enable histogram?"="button:show_histogram?") -> (w368:refnum<class "DisplayDL090216.lvclass">)
            n155 = call-dynamic "set_histogram_enabled.vi"("error in (no error)"=w377, "DisplayDL090216 in"=w368) -> ("error out"=w375:errorcluster, "DisplayDL090216 out"=w367:refnum<class "DisplayDL090216.lvclass">)  [unwired: 8 in]
            n156 = call-dynamic "checkin.vi"("error in (no error)"=w375, "GenericDisplay in"=w367) -> ("error out"=w374:errorcluster)  [unwired: 8 in, 1 out]
          }
          event Value Change {
            n157 = event-data() -> ()  [unwired: 2 out]
            n158 = Current VI's Path() -> (path=w381:path)
            n159 = call-dynamic "undock.vi"("error in (no error)"=w384, "undock?"="button:undock", "VI path"=w381, "component in"=w385) -> ("error out"=w383:errorcluster)  [unwired: 6 in, 1 out]
          }
          event Value Change {
            n160 = event-data() -> ("NewVal"=w388:T1)  [unwired: 1 out]
            n161 = case "undock main window?" shown="True" w388 {
              tunnel: w401 -> [w407 w411]
              tunnel: 0 ("Window Number (0...15)") -> [w405 w412]
              tunnel: [w406 w416] -> w391
              tunnel: [FALSE TRUE] -> w389
              frame False {
                n162 = call "IMAQ WindClose"("Window Number (0...15)"=w405, "error in (no error)"=w407) -> ("error out"=w406:errorcluster)  [unwired: 4 in]
              }
              frame True {
                w408 = TRUE ("Window is floating? (No)")
                n163 = call "IMAQ WindSetup"("Window is floating? (No)"=w408, "Window Number (0...15)"=w412, "error in (no error)"=w411, "Window has title bar? (Yes)"=w408, "Window can close? (Yes)"=FALSE, "Window can grow? (Yes)"=w408) -> ("error out"=w410:errorcluster)  [unwired: 5 in]
                n164 = local read "main display"() -> (w415:T3)
                n165 = call "IMAQ WindZoom 2"("Window Number (0...15)"=w412, "error in (no error)"=w410, "Zoom to Fit? (False)"=TRUE) -> ("error out"=w417:errorcluster)  [unwired: 5 in, 3 out]
                n166 = call "IMAQ WindDraw"("Resize to Image Size? (Y)"=TRUE, "Window Number (0...15)"=w412, "error in (no error)"=w417, "Image"=w415) -> ("error out"=w416:errorcluster)  [unwired: 6 in, 1 out]
              }
            }
            n167 = call "checkout.vi"("locked by?"="docking status", "error in (no error)"=w391) -> ("error out"=w393:errorcluster, "GenericDisplay out"=w399:refnum<class "GenericDisplay.lvclass">)  [unwired: 8 out]
            n168 = To More Specific Class(target class=w398, reference=w399, error in=w393) -> (specific class reference=w397:refnum<class "DisplayDL090216.lvclass">, error out=w394:errorcluster)
            n169 = call-dynamic "set_undocked_status.vi"("error in (no error)"=w394, "has undocked window?"=w389, "DisplayDL090216 in"=w397) -> ("error out"=w395:errorcluster, "DisplayDL090216 out"=w396:refnum<class "DisplayDL090216.lvclass">)  [unwired: 7 in]
            n170 = call-dynamic "checkin.vi"("error in (no error)"=w395, "GenericDisplay in"=w396) -> ("error out"=w392:errorcluster)  [unwired: 8 in, 1 out]
          }
          event "zero rotation button": Value Change {
            n171 = event-data() -> ()  [unwired: 2 out]
            n172 = property on="rotated by" class="DigNum (strict)"(error in=w420, "Val(Sgnl)"=dbl[unit] 0.0 ("Value (Signaling)")) -> (error out=w419:errorcluster)  [unwired: 1 in, 1 out]
          }
          event "stop": Value Change {
            n173 = event-data() -> ()  [unwired: 2 out]
            n174 = call "IMAQ WindClose"("Close All Windows (False)"=TRUE, "error in (no error)"=w426) -> ("error out"=w425:errorcluster)  [unwired: 4 in]
          }
          event "optimise", "first image received?": Value Change {
            n175 = event-data() -> ()  [unwired: 2 out]
            n176 = call "checkout.vi"("locked by?"=" \"optimise\" value change" ("string"), "error in (no error)"=w446) -> ("error out"=w443:errorcluster, "GenericDisplay out"=w444:refnum<class "GenericDisplay.lvclass">)  [unwired: 8 out]
            n177 = To More Specific Class(target class=w445, reference=w444, error in=w443) -> (specific class reference=w438:refnum<class "DisplayDL090216.lvclass">, error out=w442:errorcluster)
            n178 = Unbundle By Name(w438) -> ("range/offset processor"=w440:refnum<class "ImageProcessorDL090216RangeOffset.lvclass">)
            n179 = call-dynamic "optimise.vi"("error in (no error)"=w442, "DL090216RangeOffsetImageProcessor in"=w440) -> ("error out"=w449:errorcluster, "DL090216RangeOffsetImageProcessor out"=w448:refnum<class "ImageProcessorDL090216RangeOffset.lvclass">)  [unwired: 8 out]
            n180 = call-dynamic "get_master_range_offset.vi"("error in (no error)"=w449, "DL090216RangeOffsetImageProcessor.lvclass in"=w448) -> ("error out"=w441:errorcluster, "master"=w447:T5, "DL090216RangeOffsetImageProcessor.lvclass out"=w439:refnum<class "ImageProcessorDL090216RangeOffset.lvclass">)  [unwired: 7 out]
            n181 = local write "master range and offset"(w447) -> ()
            n182 = Bundle By Name(cluster=w438, "range/offset processor"=w439) -> (w437:refnum<class "DisplayDL090216.lvclass">)
            n183 = call-dynamic "checkin.vi"("error in (no error)"=w441, "GenericDisplay in"=w437) -> ("error out"=w432:errorcluster)  [unwired: 8 in, 1 out]
            n184 = Scan From String(input string="process", error in=w432, default 1=action_enum."process" ("trigger")) -> (error out=w431:errorcluster, output 1=w430:T4)  [unwired: 2 in, 2 out]
          }
          event Value Change {
            n185 = event-data() -> ()  [unwired: 2 out]
            n186 = call-dynamic "clear.vi"("error in (no error)"=w453, "DL090216RangeOffsetImageProcessor in"=w454) -> ("error out"=w457:errorcluster, "DL090216RangeOffsetImageProcessor out"=w456:refnum<class "ImageProcessorDL090216RangeOffset.lvclass">)  [unwired: 8 out]
            n187 = call-dynamic "set_master_range_offset.vi"("error in (no error)"=w457, "range and offset"="master range and offset", "DL090216RangeOffsetImageProcessor.lvclass in"=w456) -> ("error out"=w461:errorcluster, "DL090216RangeOffsetImageProcessor.lvclass out"=w455:refnum<class "ImageProcessorDL090216RangeOffset.lvclass">)  [unwired: 7 out]
            n188 = To More Generic Class(target class=refnum<class "GenericImageProcessor.lvclass"> refnum ("GenericImageProcessor.lvclass"), reference=w455) -> (generic class reference=w459:refnum<class "GenericImageProcessor.lvclass">)
            n189 = call-dynamic "send_image_processor_update.vi"("error in (no error)"=w461, "image processor update"=w459, "DL090216Display in"=w458) -> ("error out"=w452:errorcluster)  [unwired: 8 out]
          }
          event "channel colours": Value Change {
            w479 = T9[] [] items=["none", "red", "green", "blue", "grey scale", "custom"] ("channel colours")
            n190 = event-data() -> ("OldVal"=w472:T6[], "NewVal"=w471:T6[])  [unwired: 1 out]
            n191 = call "verify_new_color_channel.vi"("error in (no error)"=w474, "channel colours new"=w471, "channel colours old"=w472) -> ("error out"=w473:errorcluster, "channel colours out"=w469:T6[])  [unwired: 7 in]
            n192 = call "checkout.vi"("locked by?"="\"channel colours\" value change", "error in (no error)"=w473) -> ("error out"=w482:errorcluster, "GenericDisplay out"=w481:refnum<class "GenericDisplay.lvclass">)  [unwired: 8 out]
            n193 = To More Specific Class(target class=w475, reference=w481, error in=w482) -> (specific class reference=w484:refnum<class "DisplayDL090216.lvclass">, error out=w480:errorcluster)
            n194 = Type Cast(type=w479, x=w469) -> (*(type *) &x=w478:T9[])
            n195 = call-dynamic "set_channel_colours.vi"("error in (no error)"=w480, "channel colours"=w478, "DL090216Display.lvclass in"=w484) -> ("error out"=w483:errorcluster, "DL090216Display.lvclass out"=w485:refnum<class "DisplayDL090216.lvclass">)  [unwired: 7 out]
            n196 = call-dynamic "checkin.vi"("error in (no error)"=w483, "GenericDisplay in"=w485) -> ("error out"=w470:errorcluster)  [unwired: 8 in, 1 out]
            n197 = property on="channel colours" class="Arr (strict)"(error in=w470, "Value"=w469) -> (error out=w466:errorcluster)  [unwired: 1 in, 1 out]
            n198 = Scan From String(input string="process", error in=w466, default 1=action_enum."process" ("trigger")) -> (error out=w465:errorcluster, output 1=w464:T4)  [unwired: 2 in, 2 out]
          }
          event "flipped?", "rotated by", "x scaling": Value Change {
            n199 = event-data() -> ()  [unwired: 2 out]
            n200 = call "checkout.vi"("locked by?"="flipped/rotation angle: value change " ("string"), "error in (no error)"=w500) -> ("error out"=w502:errorcluster, "GenericDisplay out"=w501:refnum<class "GenericDisplay.lvclass">)  [unwired: 8 out]
            n201 = To More Specific Class(target class=refnum<class "DisplayDL090216.lvclass"> refnum ("DL090216Display.lvclass"), reference=w501, error in=w502) -> (specific class reference=w499:refnum<class "DisplayDL090216.lvclass">, error out=w496:errorcluster)
            n202 = Bundle By Name(cluster=w499, "x scaling"="x scaling", "flip image?"="flipped?", "rotation angle"="rotated by") -> (w497:refnum<class "DisplayDL090216.lvclass">)
            n203 = call-dynamic "checkin.vi"("error in (no error)"=w496, "GenericDisplay in"=w497) -> ("error out"=w489:errorcluster)  [unwired: 8 in, 1 out]
            n204 = Scan From String(input string="process", error in=w489, default 1=action_enum."process" ("trigger")) -> (error out=w488:errorcluster, output 1=w487:T4)  [unwired: 2 in, 2 out]
          }
          event "averaging": Value Change {
            n205 = event-data() -> ("CtlRef"=w517:refnum<vi>)  [unwired: 1 out]
            n206 = property class="DigNum (strict)"(reference=w517, error in=w516) -> (error out=w513:errorcluster, "Label.Text"=w512:string)  [unwired: 1 out]
            n207 = call "checkout.vi"("locked by?"=w512, "error in (no error)"=w513) -> ("error out"=w515:errorcluster, "GenericDisplay out"=w514:refnum<class "GenericDisplay.lvclass">)  [unwired: 8 out]
            n208 = To More Specific Class(target class=w508, reference=w514, error in=w515) -> (specific class reference=w507:refnum<class "DisplayDL090216.lvclass">, error out=w511:errorcluster)
            n209 = Bundle By Name(cluster=w507, "averaging"="averaging") -> (w505:refnum<class "DisplayDL090216.lvclass">)
            n210 = call-dynamic "checkin.vi"("error in (no error)"=w511, "GenericDisplay in"=w505) -> ("error out"=w510:errorcluster)  [unwired: 8 in, 1 out]
          }
          event "enable scale bar?": Value Change {
            n211 = event-data() -> ("CtlRef"=w522:refnum<vi>)  [unwired: 1 out]
            n212 = property class="Bool (strict)"(reference=w522, error in=w521) -> (error out=w520:errorcluster, "Label.Text"=w519:string)  [unwired: 1 out]
            n213 = call "checkout.vi"("locked by?"=w519, "error in (no error)"=w520) -> ("error out"=w536:errorcluster, "GenericDisplay out"=w537:refnum<class "GenericDisplay.lvclass">)  [unwired: 8 out]
            n214 = To More Specific Class(target class=w538, reference=w537, error in=w536) -> (specific class reference=w535:refnum<class "DisplayDL090216.lvclass">, error out=w532:errorcluster)
            n215 = Unbundle By Name(w535) -> ("displayed image"=w530:refnum<class "Image.lvclass">)
            n216 = call "set_scale_bar_state.vi"("error in (no error)"=w532, "enable?"="enable scale bar?", "Image in"=w530) -> ("error out"=w533:errorcluster, "Image out"=w529:refnum<class "Image.lvclass">)  [unwired: 7 out]
            n217 = Bundle By Name(cluster=w535, "displayed image"=w529) -> (w534:refnum<class "DisplayDL090216.lvclass">)
            n218 = call-dynamic "checkin.vi"("error in (no error)"=w533, "GenericDisplay in"=w534) -> ("error out"=w525:errorcluster)  [unwired: 8 in, 1 out]
            n219 = Scan From String(input string="process", error in=w525, default 1=action_enum."process" ("trigger")) -> (error out=w524:errorcluster, output 1=w523:T4)  [unwired: 2 in, 2 out]
          }
          event "enable x middle line?", "enable y middle line?": Value Change {
            n220 = event-data() -> ()  [unwired: 2 out]
            n221 = call "checkout.vi"("locked by?"="\"enable middle x/y line?\" value change" ("string"), "error in (no error)"=w555) -> ("error out"=w557:errorcluster, "GenericDisplay out"=w556:refnum<class "GenericDisplay.lvclass">)  [unwired: 8 out]
            n222 = To More Specific Class(target class=w554, reference=w556, error in=w557) -> (specific class reference=w553:refnum<class "DisplayDL090216.lvclass">, error out=w550:errorcluster)
            n223 = Unbundle By Name(w553) -> ("displayed image"=w546:refnum<class "Image.lvclass">)
            n224 = call "set_middle_line_states.vi"("error in (no error)"=w550, "draw y line?"="enable y middle line?", "draw x line?"="enable x middle line?", "Image in"=w546) -> ("error out"=w551:errorcluster, "Image out"=w547:refnum<class "Image.lvclass">)  [unwired: 6 out]
            n225 = Bundle By Name(cluster=w553, "displayed image"=w547) -> (w552:refnum<class "DisplayDL090216.lvclass">)
            n226 = call-dynamic "checkin.vi"("error in (no error)"=w551, "GenericDisplay in"=w552) -> ("error out"=w542:errorcluster)  [unwired: 8 in, 1 out]
            n227 = Scan From String(input string="process", error in=w542, default 1=action_enum."process" ("trigger")) -> (error out=w541:errorcluster, output 1=w540:T4)  [unwired: 2 in, 2 out]
          }
          event "adjust range/offset button": Value Change {
            n228 = event-data() -> ()  [unwired: 2 out]
            n229 = call "obtain_latest_instance.vi"("error in (no error)"=w568) -> ("error out"=w567:errorcluster, "GenericDisplay out"=w566:refnum<class "GenericDisplay.lvclass">)  [unwired: 1 in, 8 out]
            n230 = To More Specific Class(target class=w571, reference=w566, error in=w567) -> (specific class reference=w570:refnum<class "DisplayDL090216.lvclass">, error out=w572:errorcluster)
            n231 = Unbundle By Name(w570) -> ("range/offset processor"=w569:refnum<class "ImageProcessorDL090216RangeOffset.lvclass">)
            n232 = call-dynamic "adjust.vi"("error in (no error)"=w572, "DL090216RangeOffsetImageProcessor in"=w569) -> ("error out"=w562:errorcluster)  [unwired: 9 out]
            n233 = Scan From String(input string="process", error in=w562, default 1=action_enum."process" ("trigger")) -> (error out=w561:errorcluster, output 1=w560:T4)  [unwired: 2 in, 2 out]
          }
        }
        n234 = call-dynamic "send_internal_trigger.vi"("unique insertion?"=w229, "error in (no error)"=w231, "trigger"=w223, "DL090216Display in"=w228) -> ("error out"=w227:errorcluster, "DL090216Display out"=w230:refnum<class "DisplayDL090216.lvclass">)  [unwired: 6 out]
        "event handling loop error" <- w227
        n235 = Unbundle By Name(w227) -> ("status"=w226:bool)
        n236 = Or(x=w226, y=w225) -> (x .or. y?=w224:bool)
        "event handling loop counter" <- w234
      }
      n237 = property on="stop" class="Bool (strict)"("Val(Sgnl)"=w57) -> ()  [unwired: 2 in, 2 out]
      n238 = call-dynamic "flush_trigger_queue.vi"("error in (no error)"=w42, "GenericToplevelComponent in"=w40) -> ("error out"=w39:errorcluster, "GenericToplevelComponent out"=w41:refnum<class "DisplayDL090216.lvclass">)  [unwired: 8 in]
      n239 = call "send_error.vi"("additional message"="Error after statemachine loop!", "error in (no error)"=w32) -> ("error out"=w47:errorcluster)  [unwired: 9 in]
      n240 = call "send_error.vi"("additional message"="Error after event loop!", "error in (no error)"=w39) -> ("error out"=w45:errorcluster)  [unwired: 9 in]
      n241 = Merge Errors(w45, w47) -> (w58:errorcluster)
      n242 = call "checkout.vi"("locked by?"="", "error in (no error)"=w58) -> ("error out"=w43:errorcluster)  [unwired: 9 out]
    }
    frame Error {
    }
  }
  "error out" <- w25
  "DL090216Display out" <- w24
